vi "Close.vi"(8 "error in (no error)":errorcluster, 11 "Data in":refnum<class "UI-Bus_ComplexDouble.lvclass">) -> (0 "error out":errorcluster, 3 "Data out":refnum<class "UI-Bus_ComplexDouble.lvclass">)   [LabVIEW 2021, in "UI-Bus_ComplexDouble.lvclass"]
doc: "Abstract Data Classes 2.1.1.13\nTim Streeter - TSA\nCopyright (c) 2025, TSA"
uses:
  UI-Bus_ComplexDouble.lvclass
  UI-Bus_ComplexDouble.lvclass/UI-Bus_ComplexDouble.ctl
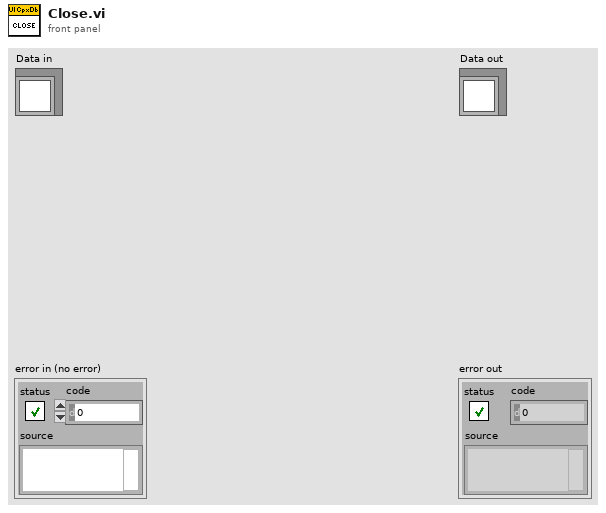
[diagram p1: front panel]
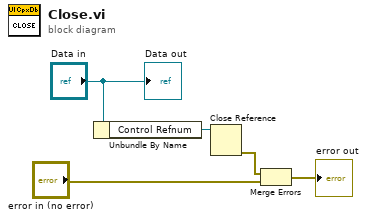
[diagram p0: block diagram]
diagram:
  n1 = Unbundle By Name("Data in") -> ("Control Refnum"=w5:refnum<vi>)
  n2 = Close Reference(reference=w5) -> (error out=w4:errorcluster)  [unwired: 1 in]
  n3 = Merge Errors(w4, "error in (no error)") -> (→"error out":errorcluster)
  "Data out" <- "Data in"
